vi "Push Stream.vi"(8 "error in (no error)":errorcluster, 10 "action":T1={"Name"=enum."Drive Left", "Priority"=0, "Data"=variant}, 11 "stream in":refnum<queue>) -> (0 "error out":errorcluster, 3 "stream out":refnum<queue>)   [LabVIEW 2015, in "Sprocket.lvlib"]
uses:
  lib/Sprocket.lvlib
  Action/Action.ctl
  Action/Action Name.ctl
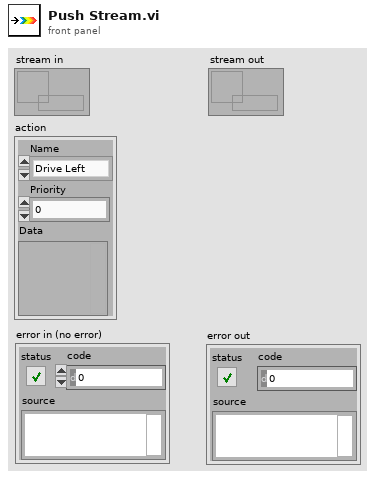
[diagram p1: front panel]
types:
  T1 = typedef "Sprocket.lvlib/Action.ctl" = cluster{"Name":T2, "Priority":i32, "Data":variant}
  T2 = typedef "Sprocket.lvlib/Action Name.ctl" = enum16{"No Action", "Drive Left", "Drive Right"}
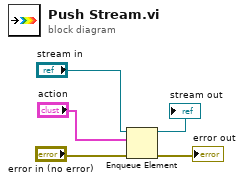
[diagram p0: block diagram]
diagram:
  n1 = Enqueue Element(queue="stream in", element="action", error in (no error)="error in (no error)") -> (queue out=→"stream out":refnum<queue>, error out=→"error out":errorcluster)  [unwired: 1 in, 1 out]
